vi "Write Upper Limit.vi"(8 "error in (no error)":errorcluster, 10 "Abs_Numeric.lvclass":refnum<class "Abs_Numeric.lvclass">, 11 "Test Numeric in":refnum<class "Test Numeric.lvclass">) -> (0 "error out":errorcluster, 3 "Test Numeric out":refnum<class "Test Numeric.lvclass">)   [LabVIEW 2021, in "BT.lvlib" / "Test Numeric.lvclass"]
uses:
  Test Numeric.lvclass
  Test Numeric.lvclass/Test Numeric.ctl
  GitHub/LV_Abstract/Source/Abs_Types/Numeric/Abs_Numeric.lvclass
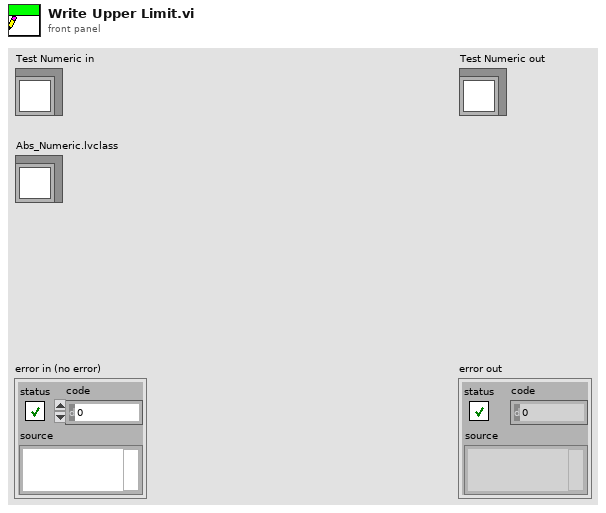
[diagram p1: front panel]
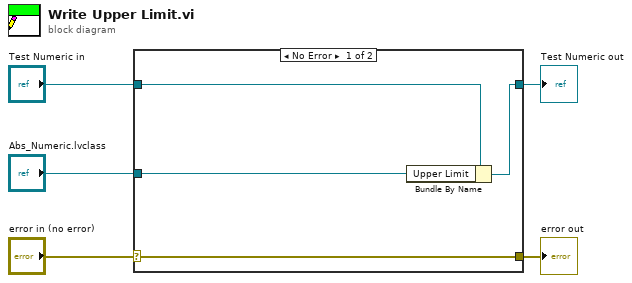
[diagram p0: block diagram]
diagram:
  n1 = case shown="No Error" "error in (no error)" {
    selector: "error in (no error)" -> [w9 w10]
    tunnel: [w9 w10] -> w4
    tunnel: [w7 w11] -> w2
    tunnel: "Test Numeric in" -> [w8 w11]
    tunnel: "Abs_Numeric.lvclass" -> [w6 _]
    frame No Error {
      n2 = Bundle By Name(cluster=w8, "Upper Limit"=w6) -> (w7:refnum<class "Test Numeric.lvclass">)
    }
    frame Error {
    }
  }
  "error out" <- w4
  "Test Numeric out" <- w2
